vi "LabVIEW Error.vi"(11 "ErrorOrSuccess JSON in":refnum<class "ErrorOrSuccess JSON.lvclass">) -> (2 "Associated LabVIEW Error":errorcluster, 3 "ErrorOrSuccess JSON out":refnum<class "ErrorOrSuccess JSON.lvclass">)   [LabVIEW 2020, in "wamplv.lvlib" / "ErrorOrSuccess JSON.lvclass"]
uses:
  ErrorOrSuccess JSON.lvclass
  ErrorOrSuccess JSON.lvclass/ErrorOrSuccess JSON.ctl
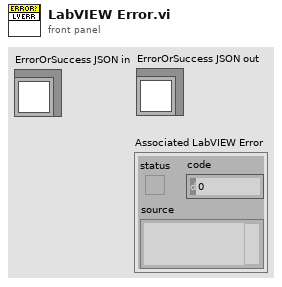
[diagram p1: front panel]
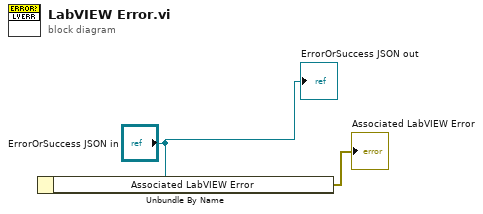
[diagram p0: block diagram]
diagram:
  n1 = Unbundle By Name("ErrorOrSuccess JSON in") -> ("Associated LabVIEW Error"=→"Associated LabVIEW Error":errorcluster)
  "ErrorOrSuccess JSON out" <- "ErrorOrSuccess JSON in"
